vi "Auto-Place lvl 3.vi"   [LabVIEW 2018]
uses:
  Implementation/Drive Operations.ctl
  Elevator/Implementation/Infrastructure/Positions.ctl
  <vilib>/Rock Robotics/Network Tables/NT Read Number.vi
  Framework/Robot Global Data.vi
types:
  T1 = cluster{"Reverse (T) / Normal (F)":bool, "Power Scaling (1=Normal) ":dbl, "Deadband Value":dbl}
  T2 = typedef "Drive Operations.ctl" = enum16{"Reserve", "Read Current", "Immediate", "J-Turn", "Play Back From Log", "Auto-Align"}
  T3 = typedef "Positions.ctl" = enum16{"MANUAL", "Bottom Pannel", "Bottom Cargo", "Feeder Station", "Cargo Ship Cargo", "Middle Pannel", "Middle Cargo", "Top Pannel", "Top Cargo"}
  T4 = typedef "Command Status Info.ctl" = cluster{"Name":string, "Status":T5, "notifier out":T6}
  T5 = typedef "Completion Status.ctl" = enum16{"Successful", "Aborted", "Incomplete"}
  T6 = typedef "Completion Notifier.ctl" = refnum<notifier>
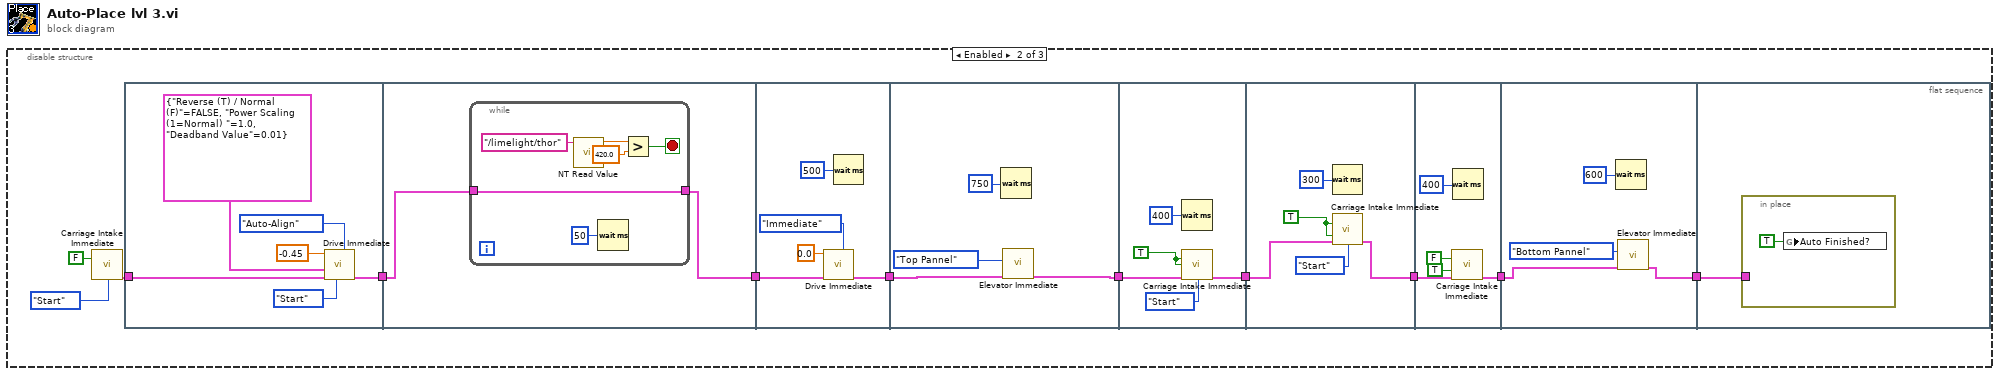
[diagram p0: block diagram]
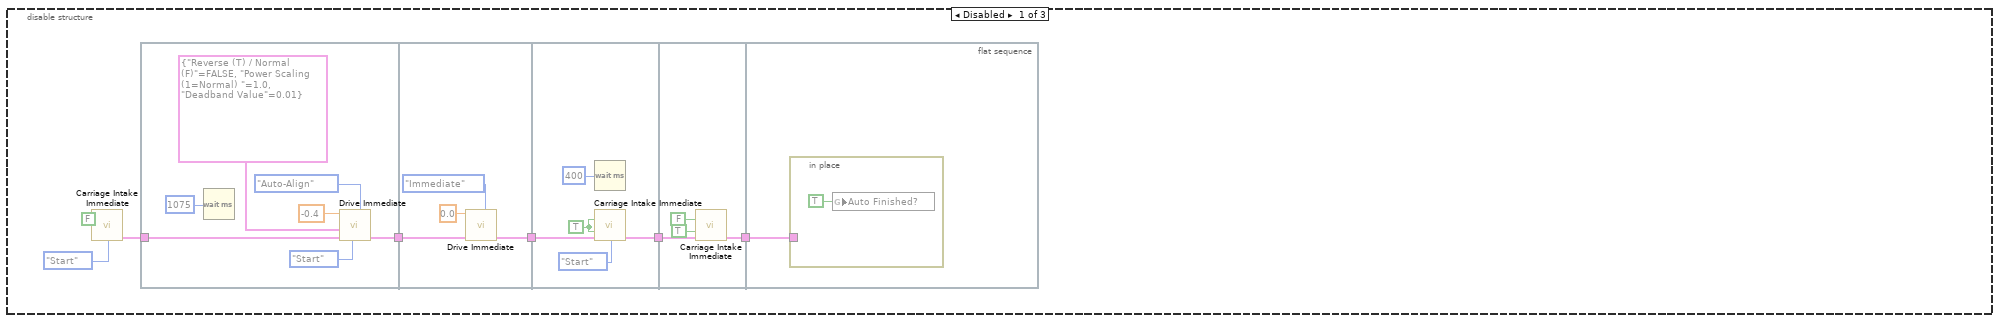
[diagram p2: hidden frame]
diagram:
  n1 = disable-structure shown="Enabled" {
    frame Disabled {
      n2 = call "Carriage Intake Immediate.vi"("Extend"=FALSE, "Synchronication"=enum16{"Start", "Wait"}."Start") -> ("Command Info Out"=w3:T4)  [unwired: 13 in]
      n3 = flat-sequence {
        tunnel: w3 -> [w11]
        tunnel: [w9] -> w7
        tunnel: w7 -> [w18]
        tunnel: [w17] -> w6
        tunnel: w6 -> [w23]
        tunnel: [w22] -> w5
        tunnel: w5 -> [w27]
        tunnel: [w25] -> w4
        tunnel: w4 -> [w28]
        frame #0 {
          n4 = Wait (ms)(milliseconds to wait=u32 1075) -> ()  [unwired: 1 out]
          n5 = call "Drive Immediate.vi"("Operation"=Drive_Operations."Auto-Align", "Synchronication"=enum16{"Start", "Wait"}."Start", "Command Info In"=w11, "Modifiers"=T1 {"Reverse (T) / Normal (F)"=FALSE, "Power Scaling (1=Normal) "=1.0, "Deadband Value"=0.01}, "Left Setpoint (Power)"=-0.4) -> ("Command Info Out"=w9:T4)  [unwired: 6 in]
        }
        frame #1 {
          n6 = call "Drive Immediate.vi"("Operation"=Drive_Operations."Immediate", "Command Info In"=w18, "Left Setpoint (Power)"=0.0) -> ("Command Info Out"=w17:T4)  [unwired: 8 in]
        }
        frame #2 {
          w19 = TRUE ("Extend")
          n7 = Wait (ms)(milliseconds to wait=u32 400) -> ()  [unwired: 1 out]
          n8 = call "Carriage Intake Immediate.vi"("Extend"=w19, "Close"=w19, "Command Info In"=w23, "Synchronication"=enum16{"Start", "Wait"}."Start") -> ("Command Info Out"=w22:T4)  [unwired: 11 in]
        }
        frame #3 {
          n9 = call "Carriage Intake Immediate.vi"("Extend"=FALSE, "Close"=TRUE, "Command Info In"=w27) -> ("Command Info Out"=w25:T4)  [unwired: 12 in]
        }
        frame #4 {
          n10 = in-place {
            in-place-border: w28 -> [_]
            n11 = global write "Robot Global Data.vi" "Auto Finished?"(TRUE ("Auto Finished?")) -> ()
          }
        }
      }
    }
    frame Enabled {
      n12 = call "Carriage Intake Immediate.vi"("Extend"=FALSE, "Synchronication"=enum16{"Start", "Wait"}."Start") -> ("Command Info Out"=w40:T4)  [unwired: 13 in]
      n13 = flat-sequence {
        tunnel: w40 -> [w43]
        tunnel: [w41] -> w37
        tunnel: w37 -> [w48]
        tunnel: [w47] -> w36
        tunnel: w36 -> [w59]
        tunnel: [w58] -> w33
        tunnel: w33 -> [w63]
        tunnel: [w62] -> w32
        tunnel: w32 -> [w68]
        tunnel: [w67] -> w35
        tunnel: w35 -> [w71]
        tunnel: [w70] -> w34
        tunnel: w34 -> [w78]
        tunnel: [w76] -> w31
        tunnel: w31 -> [w80]
        tunnel: [w79] -> w30
        tunnel: w30 -> [w83]
        frame #0 {
          n14 = call "Drive Immediate.vi"("Operation"=Drive_Operations."Auto-Align", "Synchronication"=enum16{"Start", "Wait"}."Start", "Command Info In"=w43, "Modifiers"=T1 {"Reverse (T) / Normal (F)"=FALSE, "Power Scaling (1=Normal) "=1.0, "Deadband Value"=0.01}, "Left Setpoint (Power)"=-0.45) -> ("Command Info Out"=w41:T4)  [unwired: 6 in]
        }
        frame #1 {
          n15 = while {
            tunnel: [w54] -> w47
            tunnel: w48 -> [w54]
            stop <- w50 stop-if-true
            n16 = call-poly <vilib>:"NT Read Value.vi"("Name"="/limelight/thor") -> ("Numeric"=w52:dbl)  [unwired: 9 in, 1 out]
            n17 = Wait (ms)(milliseconds to wait=u32 50) -> ()  [unwired: 1 out]
            n18 = Greater?(x=w52, y=420.0) -> (0:w50:bool)
          }
        }
        frame #2 {
          n19 = call "Drive Immediate.vi"("Operation"=Drive_Operations."Immediate", "Command Info In"=w59, "Left Setpoint (Power)"=0.0) -> ("Command Info Out"=w58:T4)  [unwired: 8 in]
          n20 = Wait (ms)(milliseconds to wait=u32 500) -> ()  [unwired: 1 out]
        }
        frame #3 {
          n21 = Wait (ms)(milliseconds to wait=u32 750) -> ()  [unwired: 1 out]
          n22 = call "Elevator Immediate.vi"("Command Info In"=w63, "Position"=Positions."Top Pannel") -> ("Command Info Out"=w62:T4)  [unwired: 9 in]
        }
        frame #4 {
          w64 = TRUE ("Extend")
          n23 = Wait (ms)(milliseconds to wait=u32 400) -> ()  [unwired: 1 out]
          n24 = call "Carriage Intake Immediate.vi"("Extend"=w64, "Open"=w64, "Command Info In"=w68, "Synchronication"=enum16{"Start", "Wait"}."Start") -> ("Command Info Out"=w67:T4)  [unwired: 11 in]
        }
        frame #5 {
          w69 = TRUE ("Extend")
          n25 = Wait (ms)(milliseconds to wait=u32 300) -> ()  [unwired: 1 out]
          n26 = call "Carriage Intake Immediate.vi"("Extend"=w69, "Close"=w69, "Command Info In"=w71, "Synchronication"=enum16{"Start", "Wait"}."Start") -> ("Command Info Out"=w70:T4)  [unwired: 11 in]
        }
        frame #6 {
          n27 = call "Carriage Intake Immediate.vi"("Extend"=FALSE, "Close"=TRUE, "Command Info In"=w78) -> ("Command Info Out"=w76:T4)  [unwired: 12 in]
          n28 = Wait (ms)(milliseconds to wait=u32 400) -> ()  [unwired: 1 out]
        }
        frame #7 {
          n29 = Wait (ms)(milliseconds to wait=u32 600) -> ()  [unwired: 1 out]
          n30 = call "Elevator Immediate.vi"("Command Info In"=w80, "Position"=Positions."Bottom Pannel") -> ("Command Info Out"=w79:T4)  [unwired: 9 in]
        }
        frame #8 {
          n31 = in-place {
            in-place-border: w83 -> [_]
            n32 = global write "Robot Global Data.vi" "Auto Finished?"(TRUE ("Auto Finished?")) -> ()
          }
        }
      }
    }
    frame Disabled {
    }
  }
